vi "EndOfPathHandler.vi"(6 "CurrentVel":dbl, 8 "MaxAccel":dbl, 9 "MaxVel":dbl, 10 "RobotLocation":cluster{dbl, dbl}, 11 "Path":cluster{"x":dbl, "y":dbl}[](array[cluster])=[{"x"=0.0, "y"=10.0}, {"x"=0.0, "y"=80.0}, {"x"=85.0, "y"=140.0}, {"x"=85.0, "y"=20.0}, {"x"=40.0, "y"=15.0}]) -> (0 "Done":bool, 1 "Override":bool, 2 "ExtraPowerOut":dbl, 3 "VelOut":dbl)   [LabVIEW 2016]
uses:
  <vilib>/addons/control/pid/pid.llb/PID (DBL).vi
  <vilib>/addons/control/pid/NI_PID_pid.lvlib
panel:
  in  "PID gains":T1 {"derivative time (Td, min)" format="%.3f"; "integral time (Ti, min)" format="%.3f"; "proportional gain (Kc)" format="%.3f"}
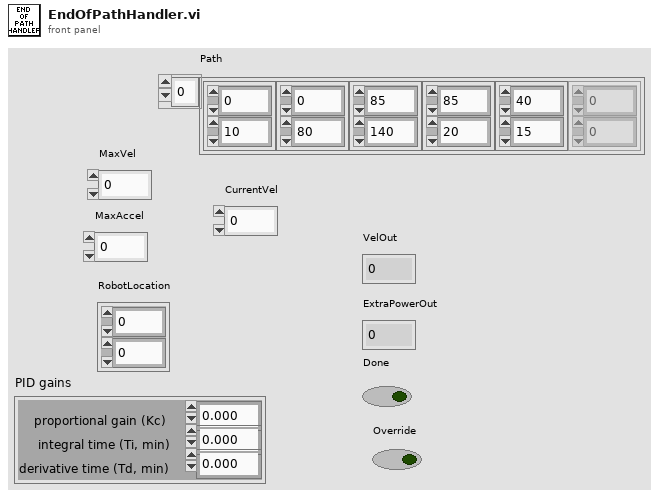
[diagram p1: front panel]
types:
  T1 = cluster{"proportional gain (Kc)":dbl, "integral time (Ti, min)":dbl, "derivative time (Td, min)":dbl}
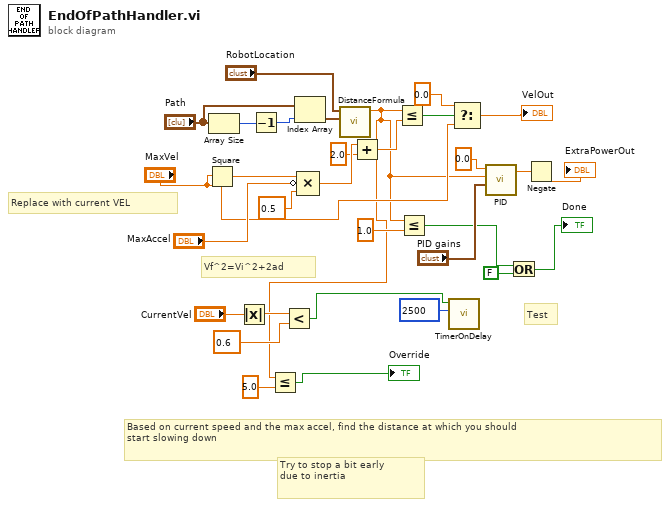
[diagram p0: block diagram]
diagram:
  # "Test"
  # "Based on current speed and the max accel, find the distance at which you should\nstart slowing down"
  # "Try to stop a bit early\ndue to inertia"
  # "Replace with current VEL"
  # "Vf^2=Vi^2+2ad"
  n1 = Square(x="MaxVel") -> (x^2=w31:dbl)
  n2 = Array Size(array="Path") -> (size(s)=w28:i32)
  n3 = Absolute Value(x="CurrentVel") -> (abs(x)=w7:dbl)
  n4 = Decrement(x=w28) -> (x-1=w27:i32)
  n5 = Less?(x=w7, y=0.6) -> (x < y?=w4:bool)
  n6 = Index Array(array="Path", index=w27) -> (element=w25:cluster{"x":dbl, "y":dbl})
  n7 = Compound Arithmetic op=MULTIPLY(w31, invert "MaxAccel", 0.5 ("value")) -> (w13:dbl)
  n8 = call "DistanceFormula.vi"("Point 2"=w25, "Point 1"="RobotLocation") -> ("Distance"=w5:dbl)  [unwired: 9 in]
  n9 = Less Or Equal?(x=w5, y=5.0) -> (x <= y?=→"Override":bool)
  n10 = Add(x=w13, y=2.0) -> (x+y=w11:dbl)
  n11 = Less Or Equal?(x=w5, y=w11) -> (x <= y?=w22:bool)
  n12 = Less Or Equal?(x=w5, y=1.0) -> (x <= y?=w10:bool)
  n13 = call "TimerOnDelay.vi"("Time Limit"=u32 2500, "Input"=w4) -> ()  [unwired: 9 in, 1 out]
  n14 = Select(t=0.0, s=w22, f="MaxVel") -> (s? t:f=→"VelOut":dbl)
  n15 = call-poly <vilib>:"PID.vi"("PID gains"="PID gains", "process variable"=w5, "setpoint"=0.0) -> ("output"=w16:dbl)  [unwired: 7 in, 1 out]
  n16 = Or(x=w10, y=FALSE) -> (x .or. y?=→"Done":bool)
  n17 = Negate(x=w16) -> (-x=→"ExtraPowerOut":dbl)
